vi "SendKeywordString.vi"(1 "String":string) -> (0 "Error":bool)   [LabVIEW 2014]
panel:
  # "This VI gets the telescope keywords and sends them to AzCamServer"
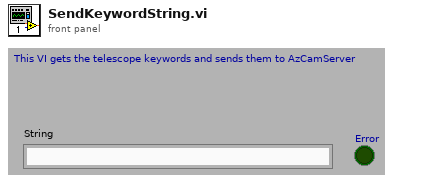
[diagram p1: front panel]
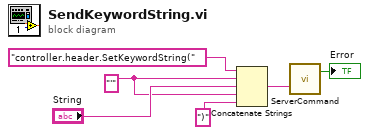
[diagram p0: block diagram]
diagram:
  w1 = "'"
  n1 = Concatenate Strings("controller.header.SetKeywordString(" ("string"), w1, "String", w1, ")" ("string")) -> (w5:string)
  n2 = call "ServerCommand.vi"("Command"=w5) -> ("Error"=→"Error":bool)  [unwired: 1 out]
